vi "Write D-Register.vi"(8 "error in":errorcluster, 9 "Data":i16, 10 "D-register number":u32=1, 11 "VISA resource name":refnum<visa-resource-name>) -> (0 "error out":errorcluster, 2 "Successfully":bool, 3 "VISA resource name out":refnum<visa-resource-name>, 4 "Responce (original)":string)   [LabVIEW 2016, in "Samwontech TEMP2xxx.lvlib"]
doc: "WSD command is used to write data to a part of D-Register by consecutive address in sequence."
uses:
  <instrlib>/Samwontech TEMP2xxx/Samwontech TEMP2xxx.lvlib
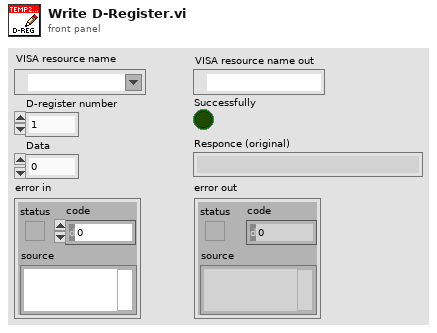
[diagram p1: front panel]
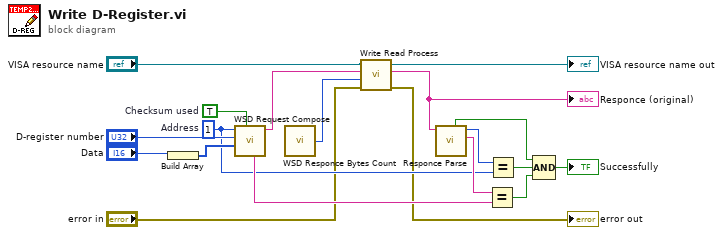
[diagram p0: block diagram]
diagram:
  w12 = u8 1  # Address
  w19 = TRUE  # Checksum used
  n1 = Build Array("Data") -> (w16:i16[])
  n2 = call <instrlib>:"WSD Request Compose.vi"("Checksum used"=w19, "Data"=w16, "D-register number"="D-register number", "Address"=w12) -> ("Request"=w1:string, "Command"=w14:string)  [unwired: 6 in]
  n3 = call <instrlib>:"WSD Responce Bytes Count.vi"() -> ("Bytes Count"=w2:u32)
  n4 = call <instrlib>:"Write Read Process.vi"("error in (no error)"="error in", "Responce Bytes Count Required"=w2, "Request"=w1, "VISA Refnum in"="VISA resource name") -> ("error out"=→"error out":errorcluster, "Responce"=w5:string, "VISA Refnum out"=→"VISA resource name out":refnum<visa-resource-name>)  [unwired: 5 in]
  "Responce (original)" <- w5
  n5 = call <instrlib>:"Responce Parse.vi"("Responce"=w5) -> ("Command"=w15:string, "Address"=w13:u8, "OK"=w9:bool)  [unwired: 6 in, 2 out]
  n6 = Equal?(x=w15, y=w14) -> (x = y?=w11:bool)
  n7 = Equal?(x=w13, y=w12) -> (x = y?=w10:bool)
  n8 = Compound Arithmetic op=AND(w9, w10, w11) -> (→"Successfully":bool)
